vi "Get Matrix - File.vi"(6 "is string":bool, 8 "error in (no error)":errorcluster, 10 "variable name":string, 11 "pipe in":T1) -> (0 "error out":errorcluster, 1 "DBL":dbl[][](array[numeric]), 3 "pipe out":T1, 4 "CDB":cdb[][](array[numeric]) format="%.2f")   [LabVIEW 2013, in "GOLPI library.lvlib"]
uses:
  GOLPI library.lvlib
  LV Process.lvlibp/Pipe Handle.ctl
  Globals.vi
  LV Process.lvlibp
panel:
  out "Array":string[](array[string])
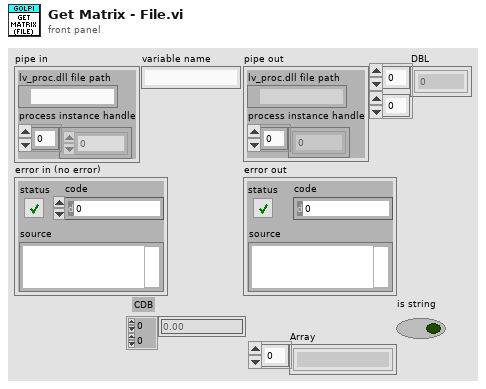
[diagram p1: front panel]
types:
  T1 = typedef "LV Process.lvlibp/Pipe Handle.ctl" = cluster{"lv_proc.dll file path":path, "process instance handle":u32[]}
  T2 = enum16{"open", "replace", "create", "open or create", "replace or create", "replace or create with confirmation"}
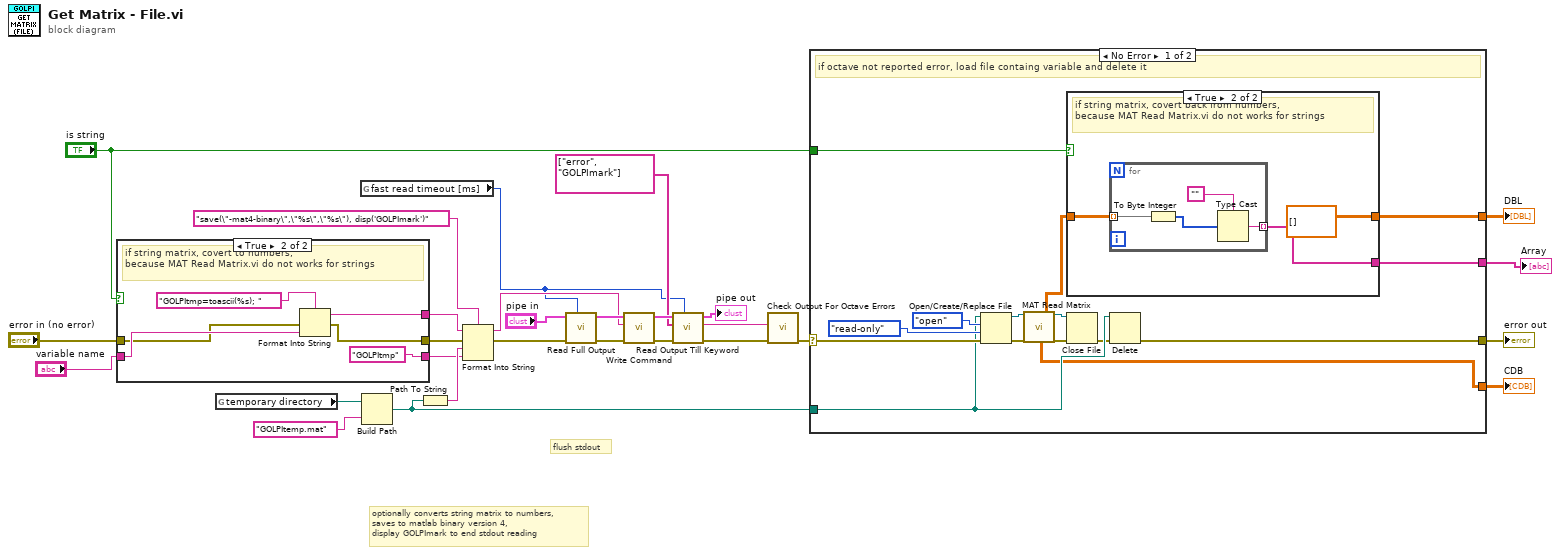
[diagram p0: block diagram]
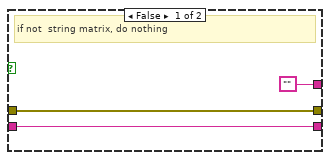
[diagram p2: hidden frame]
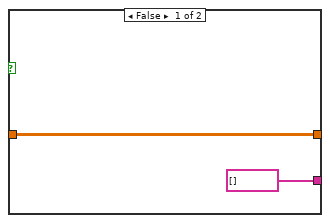
[diagram p3: hidden frame]
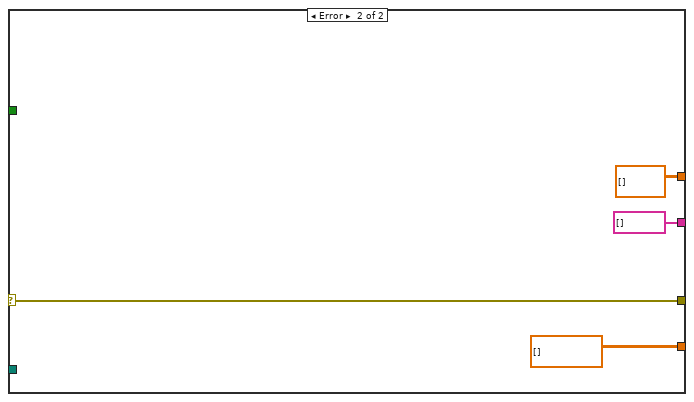
[diagram p4: hidden frame]
diagram:
  # "optionally converts string matrix to numbers,\nsaves to matlab binary version 4,\ndisplay GOLPImark to end stdout reading"
  # "flush stdout"
  n1 = case shown="True" "is string" {
    tunnel: ["" w36] -> w5
    tunnel: [w30 "GOLPItmp" ("format string")] -> w6
    tunnel: "variable name" -> [w30 w34]
    tunnel: [w29 w32] -> w4
    tunnel: "error in (no error)" -> [w29 w33]
    frame False {
      # "if not  string matrix, do nothing"
    }
    frame True {
      # "if string matrix, covert to numbers,\nbecause MAT Read Matrix.vi do not works for strings"
      n2 = Format Into String(format string="GOLPItmp=toascii(%s); ", error in=w33, w34) -> (resulting string=w36:string, error out=w32:errorcluster)  [unwired: 1 in]
    }
  }
  n3 = global read "Globals.vi" "temporary directory"() -> (w27:path)
  n4 = global read "Globals.vi" "fast read timeout [ms]"() -> (w8:u32)
  n5 = Build Path(base path=w27, name or relative path="GOLPItemp.mat") -> (appended path=w14:path)
  n6 = Path To String(path=w14) -> (string=w12:string)
  n7 = Format Into String(format string="save(\"-mat4-binary\",\"%s\",\"%s\"), disp('GOLPImark')", initial string=w5, error in=w4, w12, w6) -> (resulting string=w17:string, error out=w23:errorcluster)
  n8 = call "Read Full Output.vi"("timeout [ms]"=w8, "error in"=w23, "pipe in"="pipe in") -> ("error out"=w24:errorcluster, "pipe out"=w25:T1)  [unwired: 5 in, 2 out]
  n9 = call "Write Command.vi"("error in"=w24, "command"=w17, "pipe in"=w25) -> ("error out"=w22:errorcluster, "pipe out"=w19:T1)  [unwired: 7 in]
  n10 = call "Read Output Till Keyword.vi"("timeout [ms]"=w8, "error in"=w22, "keywords"=string[] ["error", "GOLPImark"], "pipe in"=w19) -> ("error out"=w21:errorcluster, "read buffer"=w20:string, "pipe out"=→"pipe out":T1)  [unwired: 4 in, 1 out]
  n11 = call "Check Output For Octave Errors.vi"("error in"=w21, "read buffer"=w20) -> ("error out"=w11:errorcluster)  [unwired: 9 in]
  n12 = case shown="No Error" w11 {
    selector: w11 -> [w46 w65]
    tunnel: [w43 w65] -> w28
    tunnel: [w38 string[] [] ("STR")] -> w1
    tunnel: w14 -> [w45 _]
    tunnel: [w42 cdb[][] [] ("CDB")] -> w10
    tunnel: [w39 dbl[][] [] ("DBL")] -> w9
    tunnel: "is string" -> [w41 _]
    frame No Error {
      # "if octave not reported error, load file containg variable and delete it"
      n13 = Open/Create/Replace File(file path (use dialog)=w45, error in=w46, operation (0:open)=T2."open", access (0:read/write)=enum16{"read/write", "read-only", "write-only"}."read-only") -> (refnum out=w49:refnum<file>, error out=w51:errorcluster)  [unwired: 2 in, 1 out]
      n14 = call "MAT Read Matrix.vi"("Ref Num"=w49, "Error In"=w51) -> ("CDB"=w42:cdb[][], "DBL"=w40:dbl[][], "Dup Ref Num"=w50:refnum<file>, "error out"=w52:errorcluster)  [unwired: 5 in, 9 out]
      n15 = case shown="True" w41 {
        tunnel: w40 -> [w54 w57]
        tunnel: [string[] [] w55] -> w38
        tunnel: [w54 dbl[][] [] ("DBL")] -> w39
        frame False {
        }
        frame True {
          # "if string matrix, covert back from numbers,\nbecause MAT Read Matrix.vi do not works for strings"
          n16 = for {
            tunnel: [w61] -> w55 mode=indexing
            tunnel: w57 -> [w58] mode=indexing
            n17 = To Byte Integer(number=w58) -> (8bit integer=w59:i8[])
            n18 = Type Cast(type="", x=w59) -> (*(type *) &x=w61:string)
          }
        }
      }
      n19 = Close File(refnum=w50, error in=w52) -> (error out=w44:errorcluster)  [unwired: 1 out]
      n20 = Delete(path (use dialog)=w45, error in=w44) -> (error out=w43:errorcluster)  [unwired: 3 in, 2 out]
    }
    frame Error {
    }
  }
  "error out" <- w28
  "CDB" <- w10
  "DBL" <- w9
  "Array" <- w1
